vi "Wait Sweep Waveform.vi"(8 "error in (no error)":errorcluster, 10 "Waveforms in":waveform(dbl)[](array[waveform]), 11 "Generator in":refnum<class "Generator.lvclass">) -> (0 "error out":errorcluster, 2 "Waveforms out":waveform(dbl)[](array[waveform]), 3 "Generator out":refnum<class "Generator.lvclass">)   [LabVIEW 2019, in "Generator.lvclass"]
uses:
  Generator.lvclass
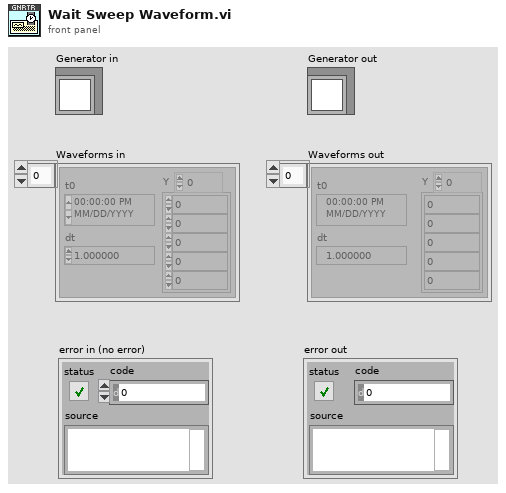
[diagram p1: front panel]
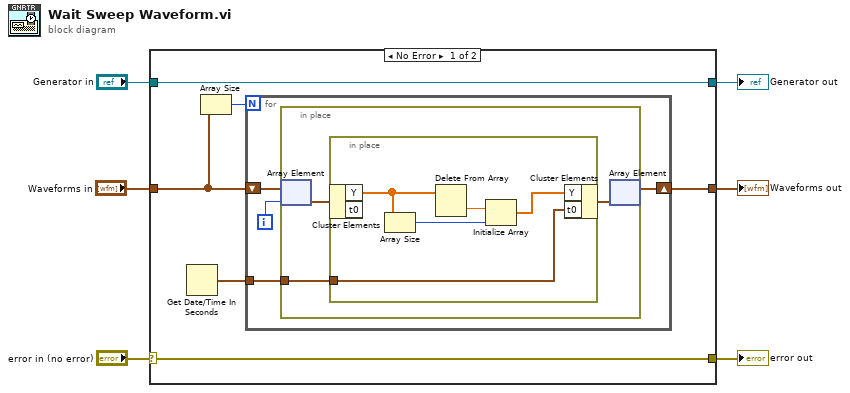
[diagram p0: block diagram]
diagram:
  n1 = case shown="No Error" "error in (no error)" {
    selector: "error in (no error)" -> [w9 w26]
    tunnel: "Generator in" -> [w8 w25]
    tunnel: [w9 w26] -> w4
    tunnel: [w8 w25] -> w3
    tunnel: "Waveforms in" -> [w11 _]
    tunnel: [w7 _] -> w1
    frame No Error {
      n2 = Get Date/Time In Seconds() -> (seconds since 1Jan1904=w12:timestamp)
      n3 = Array Size(array=w11) -> (size(s)=w10:i32)
      n4 = for {
        N: w10 -> [_]
        shift-right: [w15] -> w7
        shift-left: w11 -> [w16]
        tunnel: w12 -> [w13]
        i -> [w14]
        n5 = in-place {
          in-place-border: w13 -> [w18]
          n6 = in-place-array #1(w16, w14) -> (w19:waveform(dbl))
          n7 = in-place {
            in-place-border: w18 -> [w24]
            n8 = in-place-cluster #2(w19) -> ("Y"=w22:dbl[])  [unwired: 1 out]
            n9 = Array Size(array=w22) -> (size(s)=w23:i32)
            n10 = Delete From Array(array=w22) -> (deleted portion=w21:dbl)  [unwired: 2 in, 1 out]
            n11 = Initialize Array(w21, w23) -> (w20:dbl[])
            n12 = in-place-cluster #2("Y"=w20, "t0"=w24) -> (w17:waveform(dbl))
          }
          n13 = in-place-array #1(w17) -> (w15:waveform(dbl)[])  [unwired: 1 out]
        }
      }
    }
    frame Error {
    }
  }
  "Generator out" <- w3
  "error out" <- w4
  "Waveforms out" <- w1
